vi "Hide Animated Busy Icon with Message and Abort Button.vi"(2 "Already active? (F)":bool, 3 "Message":string, 7 "Target VI reference":refnum<vi>, 11 "Error In":errorcluster, 16 "Abort Button Name (Abort)":string="Abort", 17 "Animated Busy Icon Control Name (Animated Busy Icon)":string="Animated Busy Icon", 18 "Message Control Name (Message)":string="Message") -> (10 "Error Out":errorcluster)   [LabVIEW 2019]
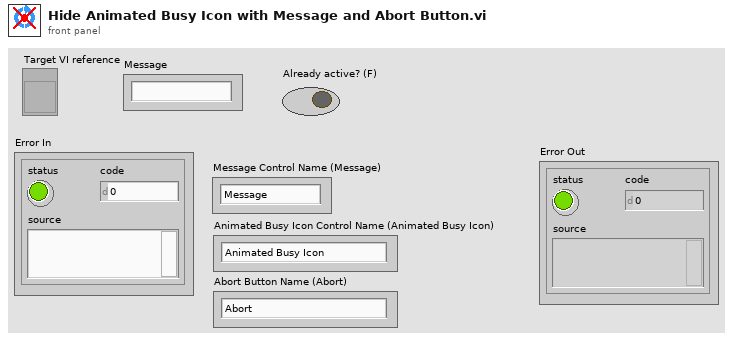
[diagram p1: front panel]
types:
  T1 = enum16{"Controls & Indicators", "Controls", "Indicators"}
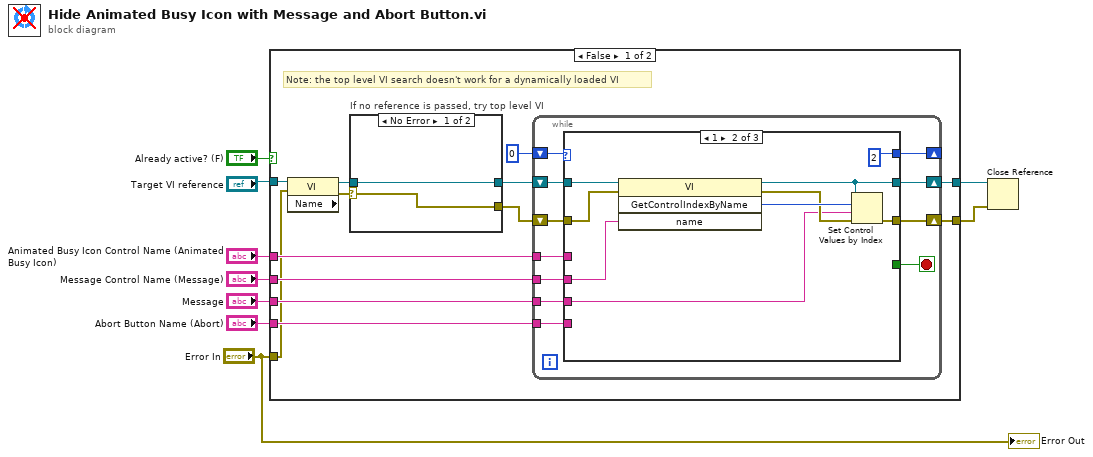
[diagram p0: block diagram]
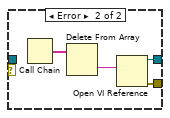
[diagram p2: hidden frame]
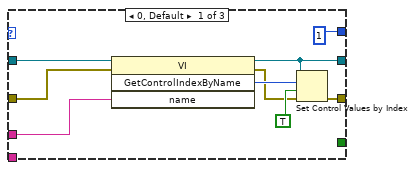
[diagram p3: hidden frame]
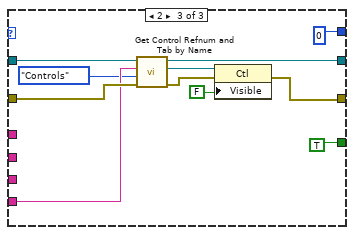
[diagram p4: hidden frame]
diagram:
  n1 = case shown="False" "Already active? (F)" {
    tunnel: [w22 w69] -> w9
    tunnel: [w21 _] -> w8
    tunnel: "Message Control Name (Message)" -> [w19 _]
    tunnel: "Animated Busy Icon Control Name (Animated Busy Icon)" -> [w18 _]
    tunnel: "Message" -> [w17 _]
    tunnel: "Target VI reference" -> [w14 w69]
    tunnel: "Abort Button Name (Abort)" -> [w11 _]
    tunnel: "Error In" -> [w10 _]
    frame False {
      # "Note: the top level VI search doesn't work for a dynamically loaded VI"
      n2 = property class="VI" props=["Name"](reference=w14, error in=w10) -> (reference out=w13:refnum<vi>, error out=w12:errorcluster)  [unwired: 1 out]
      n3 = case "If no reference is passed, try top level VI" shown="No Error" w12 {
        selector: w12 -> [w23 _]
        tunnel: [w23 w28] -> w15
        tunnel: [w24 w27] -> w16
        tunnel: w13 -> [w24 _]
        frame No Error {
        }
        frame Error {
          n4 = Call Chain() -> (call chain=w25:string[])
          n5 = Delete From Array(array=w25) -> (deleted portion=w26:string)  [unwired: 2 in, 1 out]
          n6 = Open VI Reference(vi path=w26) -> (vi reference=w27:refnum<vi>, error out=w28:errorcluster)  [unwired: 5 in]
        }
      }
      n7 = while {
        shift-right: [w36] -> w21
        shift-left: w15 -> [w39]
        shift-right: [w37] -> w22
        shift-left: w16 -> [w38]
        shift-right: [w34] -> _
        shift-left: 0 -> [w35]
        tunnel: w19 -> [w32]
        tunnel: w18 -> [w31]
        tunnel: w17 -> [w30]
        tunnel: w11 -> [w29]
        stop <- w33 stop-if-true
        n8 = case shown="1" w35 {
          tunnel: w39 -> [w45 w55 w63]
          tunnel: w38 -> [w44 w54 w64]
          tunnel: [w43 w53 w61] -> w37
          tunnel: [w42 w52 w59] -> w36
          tunnel: [1 2 0] -> w34
          tunnel: [_ _ TRUE] -> w33
          tunnel: w32 -> [_ w50 _]
          tunnel: w31 -> [w40 _ _]
          tunnel: w30 -> [_ w49 _]
          tunnel: w29 -> [_ _ w62]
          frame 0, Default {
            n9 = invoke class="VI" method="GetControlIndexByName"(reference=w44, error in=w45, "name"=w40) -> (reference out=w43:refnum<vi>, error out=w46:errorcluster, "GetControlIndexByName"=w48:i32)  [unwired: 1 in, 1 out]
            n10 = Set Control Values by Index(0:w43, 1:w48, 2:TRUE ("Visible"), 3:w46) -> (11:w42:errorcluster)
          }
          frame 1 {
            n11 = invoke class="VI" method="GetControlIndexByName"(reference=w54, error in=w55, "name"=w50) -> (reference out=w53:refnum<vi>, error out=w56:errorcluster, "GetControlIndexByName"=w57:i32)  [unwired: 1 in, 1 out]
            n12 = Set Control Values by Index(0:w53, 1:w57, 2:w49, 3:w56) -> (11:w52:errorcluster)
          }
          frame 2 {
            n13 = call "Get Control Refnum and Tab by Name.vi"("error in"=w63, "Selection"=T1."Controls", "Control Label"=w62, "VI  Ref"=w64) -> ("error out"=w65:errorcluster, "Ctl Refnum"=w66:refnum<vi>, "VI  Ref (out)"=w61:refnum<vi>)  [unwired: 3 in, 2 out]
            n14 = property class="Ctl"(reference=w66, error in=w65, "Visible"=FALSE) -> (error out=w59:errorcluster)  [unwired: 1 out]
          }
        }
      }
    }
    frame True {
    }
  }
  n15 = Close Reference(reference=w9, error in (no error)=w8) -> ()  [unwired: 1 out]
  "Error Out" <- "Error In"
